vi "Vision Processing Performance.vi"(7 "Image Size":T6=enum."320x240") -> ()   [LabVIEW 2018]
uses:
  <vilib>/Rock Robotics/WPI/Camera/WPI_CameraImageSize.ctl
  <vilib>/Rock Robotics/WPI/Camera/WPI_CameraWhite Balance Values.ctl
  <vilib>/Rock Robotics/WPI/Camera/WPI_CameraExposure Values.ctl
  <vilib>/Rock Robotics/WPI/Camera/WPI_CameraExposure Priority Values.ctl
  <vilib>/Rock Robotics/WPI/Camera/WPI_CameraFrameRate.ctl
panel:
  in  "Display Image":bool=TRUE
  out "Frames per Second":dbl format="%#.1g"
  out "Loop Time (ms)":u32
  out "Camera Image":T1(plugin-control)
  out "Color Level":i32
  out "Color Enable *":bool
  out "Exposure Priority *":T2
  out "Sharpness":i32
  out "Brightness":i32
  out "Compression *":i32
  out "Exposure":T3
  out "Exposure (%)":dbl
  out "Color Temp (K)":dbl
  out "White Balance":T4
  out "Frame Rate (fps)":T5
  out "Size W,H (pix)":cluster{i32, i32}
  out "Image Size":T6
  in  "Sharpness":i32(slide)=50 scale=0.0..100.0
  in  "Exposure Priority *":T2
  in  "Color Enable *":bool=TRUE
  in  "Color Level":i32(slide)=50 scale=0.0..100.0
  in  "Brightness":i32(slide)=50 scale=0.0..100.0
  in  "Compression *":i32(slide)=40 scale=0.0..100.0
  in  "Exposure Value":i32(slide)=33 scale=0.0..100.0
  in  "Exposure":T3=enum."Flicker-free 60 Hz"
  in  "Color Temp (K)":dbl=6000.0
  in  "Custom":cluster{"Width":i32, "Height":i32}={"Width"=320, "Height"=240}
  in  "Framerate":i32(slide)=20 scale=0.0..30.0
  in  "White Balance":T4=enum."Fixed fluorescent 1"
  # "* indicates the settings that are not supported by USB cameras"
  # "Instructions"
  # "This exmple demonstrates the reading and writing of\nall WPI camera setting. The primary and secondary\nsettings are useful for discovering how they operate on\n a given camera.\nThe initial settings section is useful for discovering\nwhat items the camera remembers and what it\nforgets across a robot reboot.\nThe example is also useful to observe how the settings\nsuch as exposure, external factors such as the amount\nof light, and viewing image displays affects framerate.\nYou may also want to open the DS to observe roboRIO\nCPU usage."
  # "Primary Settings"
  # "Secondary Settings"
  # "Initial Settings"
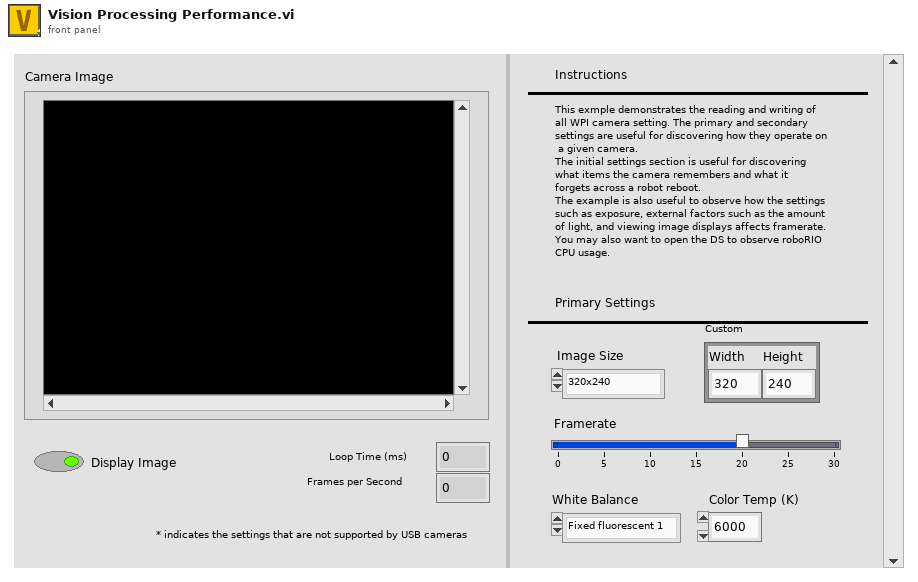
[diagram p1: front panel]
types:
  T1 = typedef "IMAQ Image.ctl" = refnum<image>
  T2 = typedef "WPI_CameraExposure Priority Values.ctl" = enum16{"None", "Prioritize frame rate", "Prioritize image quality"}
  T3 = typedef "WPI_CameraExposure Values.ctl" = enum16{"Auto", "Flicker-free 50 Hz", "Flicker-free 60 Hz", "Hold current", "Custom"}
  T4 = typedef "WPI_CameraWhite Balance Values.ctl" = enum16{"Auto", "Fixed indoor", "Fixed outdoor 1", "Fixed outdoor 2", "Fixed fluorescent 1", "Fixed fluorescent 2", "Hold current", "Custom"}
  T5 = typedef "WPI_CameraFrameRate.ctl" = u32
  T6 = typedef "WPI_CameraImageSize.ctl" = enum16{"640x480", "320x240", "160x120", "Custom"}
  T7 = typedef "Image Type" = u32
  T8 = typedef "WPI_CameraDevRef.ctl" = cluster{"Camera Address":string, "CameraStatus":errorcluster}
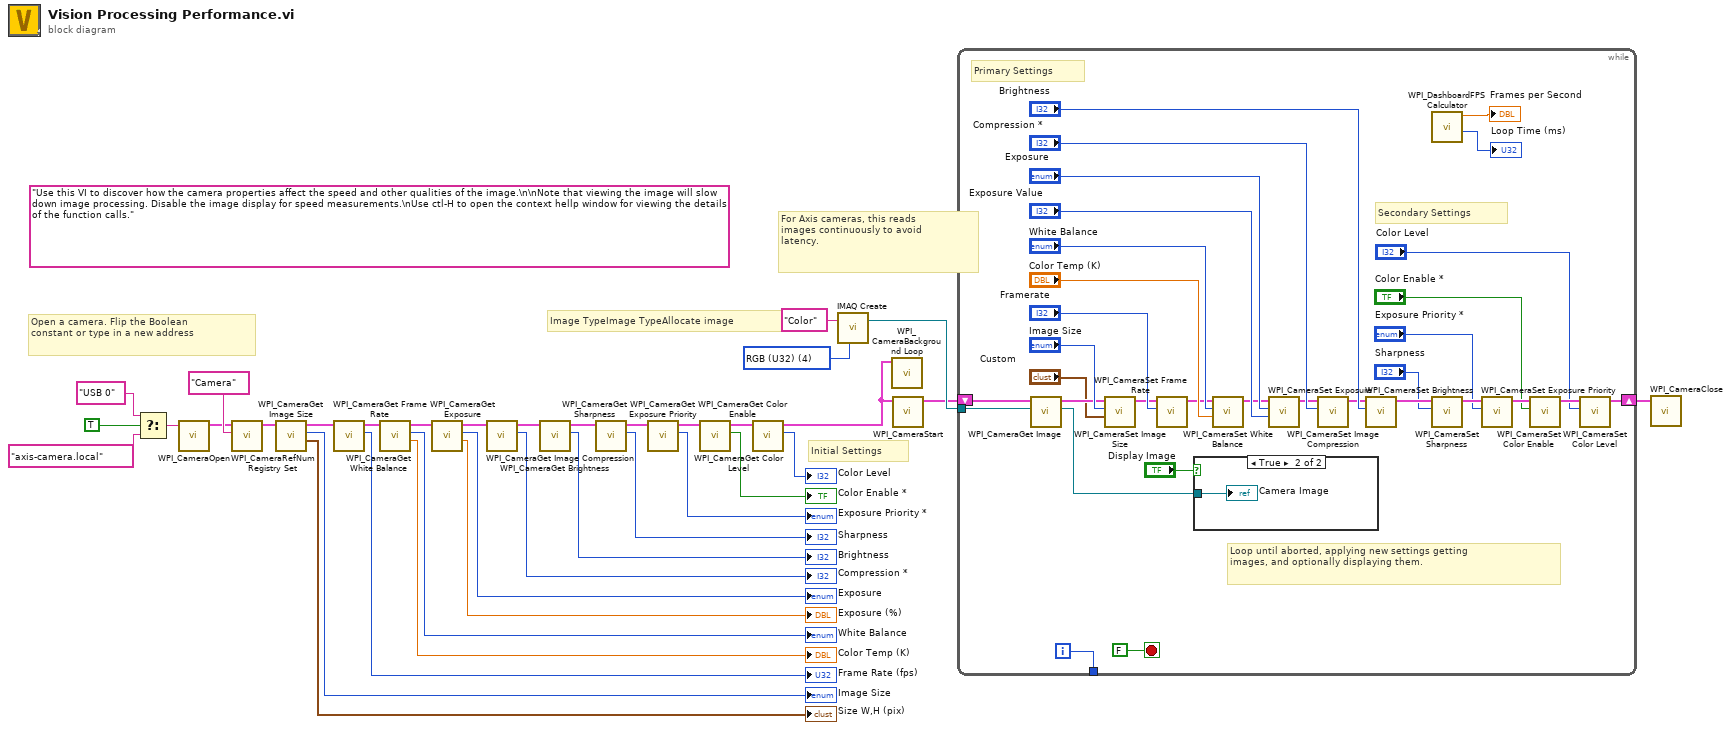
[diagram p0: block diagram]
diagram:
  (unwired) "Use this VI to discover how the camera properties affect the speed and other qualities of the image.\n\nNote that viewing the image will slow down image processing. Disable the image display for speed measurements.\nUse ctl-H to open the context hellp window for viewing the details of the function calls."
  w34 = T7 4 items=["Grayscale (U8)", "Grayscale (I16)", "Grayscale (SGL)", "Complex (CSG)", "RGB (U32)", "HSL (U32)", "RGB (U64)", "Grayscale (U16)"] ("Image Type")
  # "Initial Settings"
  # "Open a camera. Flip the Boolean\nconstant or type in a new address"
  # "For Axis cameras, this reads\nimages continuously to avoid\nlatency."
  # "Image TypeImage TypeAllocate image"
  n1 = Select(t="USB 0" ("format string"), s=TRUE ("dot notation? (F)"), f="axis-camera.local" ("format string")) -> (s? t:f=w32:string)
  n2 = call <vilib>:"WPI_CameraOpen.vi"("Camera Address"=w32) -> ("CameraDevRef"=w25:T8)  [unwired: 1 in, 9 out]
  n3 = call <vilib>:"WPI_CameraRefNum Registry Set.vi"("refnum name"="Camera", "CameraDevRef"=w25) -> ("CameraDevRef"=w24:T8)  [unwired: 2 in, 7 out]
  n4 = call <vilib>:"WPI_CameraGet Image Size.vi"("CameraDevRef"=w24) -> ("Size W,H (pix)"=→"Size W,H (pix)":cluster{i32, i32}, "Image Size"=→"Image Size":T6, "CameraDevRef Out"=w23:T8)  [unwired: 7 in, 1 out]
  n5 = call <vilib>:"WPI_CameraGet Frame Rate.vi"("CameraDevRef"=w23) -> ("Frame Rate (fps)"=→"Frame Rate (fps)":T5, "CameraDevRef Out"=w22:T8)  [unwired: 8 in, 1 out]
  n6 = call <vilib>:"WPI_CameraGet White Balance.vi"("CameraDevRef"=w22) -> ("Color Temp (K)"=→"Color Temp (K)":dbl, "White Balance"=→"White Balance":T4, "CameraDevRef Out"=w21:T8)  [unwired: 7 in, 1 out]
  n7 = call <vilib>:"WPI_CameraGet Exposure.vi"("CameraDevRef"=w21) -> ("Exposure (%)"=→"Exposure (%)":dbl, "Exposure"=→"Exposure":T3, "CameraDevRef Out"=w20:T8)  [unwired: 7 in, 1 out]
  n8 = call <vilib>:"WPI_CameraGet Image Compression.vi"("CameraDevRef"=w20) -> ("Compression"=→"Compression *":i32, "CameraDevRef Out"=w19:T8)  [unwired: 8 in, 1 out]
  n9 = call <vilib>:"WPI_CameraGet Brightness.vi"("CameraDevRef"=w19) -> ("Brightness"=→"Brightness":i32, "CameraDevRef Out"=w18:T8)  [unwired: 8 in, 1 out]
  n10 = call <vilib>:"WPI_CameraGet Sharpness.vi"("CameraDevRef"=w18) -> ("Sharpness"=→"Sharpness":i32, "CameraDevRef Out"=w17:T8)  [unwired: 8 in, 1 out]
  n11 = call <vilib>:"WPI_CameraGet Exposure Priority.vi"("CameraDevRef"=w17) -> ("Exposure Priority"=→"Exposure Priority *":T2, "CameraDevRef Out"=w16:T8)  [unwired: 8 in, 1 out]
  n12 = call <vilib>:"WPI_CameraGet Color Enable.vi"("CameraDevRef"=w16) -> ("Color Enabled"=→"Color Enable *":bool, "CameraDevRef Out"=w15:T8)  [unwired: 8 in, 1 out]
  n13 = call <vilib>:"WPI_CameraGet Color Level.vi"("CameraDevRef"=w15) -> ("Color Level"=→"Color Level":i32, "CameraDevRef Out"=w14:T8)  [unwired: 8 in, 1 out]
  n14 = call "IMAQ Create"("Image Name"="Color", "Image Type"=w34) -> ("New Image"=w33:T1)  [unwired: 2 in, 2 out]
  n15 = call <vilib>:"WPI_CameraBackground Loop.vi"("CameraDevRef"=w14) -> ()  [unwired: 11 in]
  n16 = call <vilib>:"WPI_CameraStart.vi"("CameraDevRef"=w14) -> ("CameraDevRef"=w26:T8)  [unwired: 1 in, 9 out]
  n17 = while {
    tunnel: w33 -> [w66]
    tunnel: [w65] -> _
    shift-right: [w40] -> w27
    shift-left: w26 -> [w62]
    i -> [w65]
    stop <- FALSE stop-if-true
    # "Primary Settings"
    # "Secondary Settings"
    # "Loop until aborted, applying new settings getting\nimages, and optionally displaying them."
    n18 = call <vilib>:"WPI_CameraGet Image.vi"("Image"=w66, "CameraDevRef"=w62) -> ("Image Out"=w63:T1, "CameraDevRef Out"=w56:T8)  [unwired: 7 in, 1 out]
    n19 = call <vilib>:"WPI_CameraSet Image Size.vi"("Size W,H (pix)"="Custom", "Image Size"="Image Size", "CameraDevRef"=w56) -> ("CameraDevRef Out"=w51:T8)  [unwired: 1 in, 7 out]
    n20 = call <vilib>:"WPI_CameraSet Frame Rate.vi"("Frame Rate (fps)"="Framerate", "CameraDevRef"=w51) -> ("CameraDevRef Out"=w50:T8)  [unwired: 1 in, 8 out]
    n21 = case shown="True" "Display Image" {
      tunnel: w63 -> [_ w68]
      frame False {
      }
      frame True {
        "Camera Image" <- w68
      }
    }
    n22 = call <vilib>:"WPI_CameraSet White Balance.vi"("Color Temp (K)"="Color Temp (K)", "White Balance"="White Balance", "CameraDevRef"=w50) -> ("CameraDevRef Out"=w47:T8)  [unwired: 1 in, 7 out]
    n23 = call <vilib>:"WPI_CameraSet Exposure.vi"("Exposure (%)"="Exposure Value", "Exposure"="Exposure", "CameraDevRef"=w47) -> ("CameraDevRef Out"=w49:T8)  [unwired: 1 in, 7 out]
    n24 = call <vilib>:"WPI_CameraSet Image Compression.vi"("Compression"="Compression *", "CameraDevRef"=w49) -> ("CameraDevRef Out"=w48:T8)  [unwired: 1 in, 8 out]
    n25 = call <vilib>:"WPI_CameraSet Brightness.vi"("Brightness"="Brightness", "CameraDevRef"=w48) -> ("CameraDevRef Out"=w44:T8)  [unwired: 2 in, 7 out]
    n26 = call <vilib>:"WPI_DashboardFPS Calculator.vi"() -> ("delta (ms)"=→"Loop Time (ms)":u32, "fps"=→"Frames per Second":dbl)  [unwired: 10 in]
    n27 = call <vilib>:"WPI_CameraSet Sharpness.vi"("Sharpness"="Sharpness", "CameraDevRef"=w44) -> ("CameraDevRef Out"=w43:T8)  [unwired: 8 in, 1 out]
    n28 = call <vilib>:"WPI_CameraSet Exposure Priority.vi"("Exposure Priority"="Exposure Priority *", "CameraDevRef"=w43) -> ("CameraDevRef Out"=w42:T8)  [unwired: 8 in, 1 out]
    n29 = call <vilib>:"WPI_CameraSet Color Enable.vi"("Color Enabled"="Color Enable *", "CameraDevRef"=w42) -> ("CameraDevRef Out"=w41:T8)  [unwired: 8 in, 1 out]
    n30 = call <vilib>:"WPI_CameraSet Color Level.vi"("Color Level"="Color Level", "CameraDevRef"=w41) -> ("CameraDevRef Out"=w40:T8)  [unwired: 8 in, 1 out]
  }
  n31 = call <vilib>:"WPI_CameraClose.vi"("CameraDevRef"=w27) -> ()  [unwired: 1 in, 10 out]
